vi "AlliGator Phasor Plot Image Edit ROI Name.vi"(11 "ROI Name in":string) -> (0 "accepted?":bool, 2 "Old ROI Name":string, 3 "ROI Name out":string)   [LabVIEW 2021, in "AlliGator ROIs.lvlib"]
doc: "Changes current Phasor Plot image ROI name."
uses:
  AlliGator ROIs.lvlib
  AlliGator ROI Manager Actions.ctl
  AlliGator Phasor Plot Image ROI Storage [SGL] v3.vi
panel:
  # "see the AlliGator License on the block diagram (Ctrl+E or Window:Show Block Diagram)"
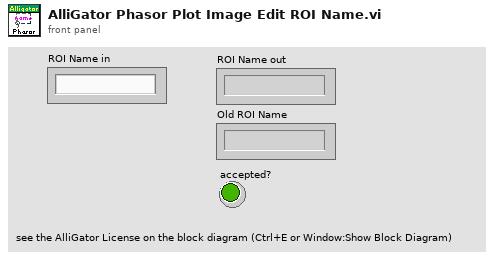
[diagram p1: front panel]
types:
  T1 = typedef "AlliGator ROIs.lvlib/AlliGator ROI Manager Actions.ctl" = enum16{"Undefined", "Delete Current ROI", "Delete All Unselected ROIs", "Delete Multiple ROIs", "Delete All ROIs", "Swap ROIs", "Insert ROI", "Update Current ROI Descriptor", "Rename Current ROI", "Store New ROI", "Store Multiple ROIs", "Select Next ROI", "Select Previous ROI", "Find Selected ROI", "Show All ROIs", "Update ROI Manager Window", "Merge All ROIs", "Unmerge ROI", "Set Selected ROI by ID"}
  T2 = typedef "ROI Descriptor" = cluster{"Global Rectangle":i32[], "Contours":cluster{"ID":enum32{"External", "Internal"}, "Type":u32, "Coordinates":i32[]}[]}
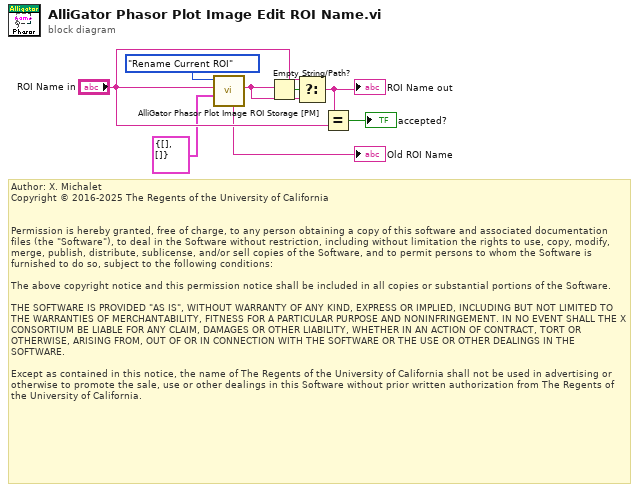
[diagram p0: block diagram]
diagram:
  # "Author: X. Michalet\nCopyright © 2016-2025 The Regents of the University of California\n \n\nPermission is hereby granted, free of charge, to any person obtaining a copy of this software and associated documentation files (the \"Software\"), to deal in the Software without restriction, including without limitation the rights to use, copy, modify, merge, publish, distribute, sublicense, and/or sell copies of the Software, and to permit persons to whom the Software is furnished to do so, subject to the following conditions:\n\nThe above copyright notice and this permission notice shall be included in all copies or substantial portions of the Software.\n\nTHE SOFTWARE IS PROVIDED \"AS IS\", WITHOUT WARRANTY OF ANY KIND, EXPRESS OR IMPLIED, INCLUDING BUT NOT LIMITED TO THE WARRANTIES OF MERCHANTABILITY, FITNESS FOR A PARTICULAR PURPOSE AND NONINFRINGEMENT. IN NO EVENT SHALL THE X CONSORTIUM BE LIABLE FOR ANY CLAIM, DAMAGES OR OTHER LIABILITY, WHETHER IN AN ACTION OF CONTRACT, TORT OR OTHERWISE, ARISING FROM, OUT OF OR IN CONNECTION WITH THE SOFTWARE OR THE USE OR OTHER DEALINGS IN THE SOFTWARE.\n\nExcept as contained in this notice, the name of The Regents of the University of California shall not be used in advertising or otherwise to promote the sale, use or other dealings in this Software without prior written authorization from The Regents of the University of California."
  n1 = call-poly "AlliGator Phasor Plot Image ROI Storage [PM].vi"("Current ROI Descriptor"=T2 {"Global Rectangle"=[], "Contours"=[]}, "Default Name (\"ROI\")"="ROI Name in", "Action"=AlliGator_ROI_Manager_Actions."Rename Current ROI") -> ("Current ROI Name"=w3:string, "Old ROI Name"=→"Old ROI Name":string)  [unwired: 3 in, 4 out]
  n2 = Empty String/Path?(string/path=w3) -> (empty?=w7:bool)
  n3 = Select(t="ROI Name in", s=w7, f=w3) -> (s? t:f=w6:string)
  "ROI Name out" <- w6
  n4 = Equal?(x=w6, y="ROI Name in") -> (x = y?=→"accepted?":bool)
